vi "Probability Bar.vi"(7 "QuWire in":refnum<class "QuWire.lvclass">) -> (4 "Porababilities":dbl[](array[numeric]), 15 "Qubits n":i32)   [LabVIEW 2020]
uses:
  QuSim/QuWire/QuWire.lvclass
panel:
  out "Probability Bar Graph":cluster{i32[], dbl[]}(graph)
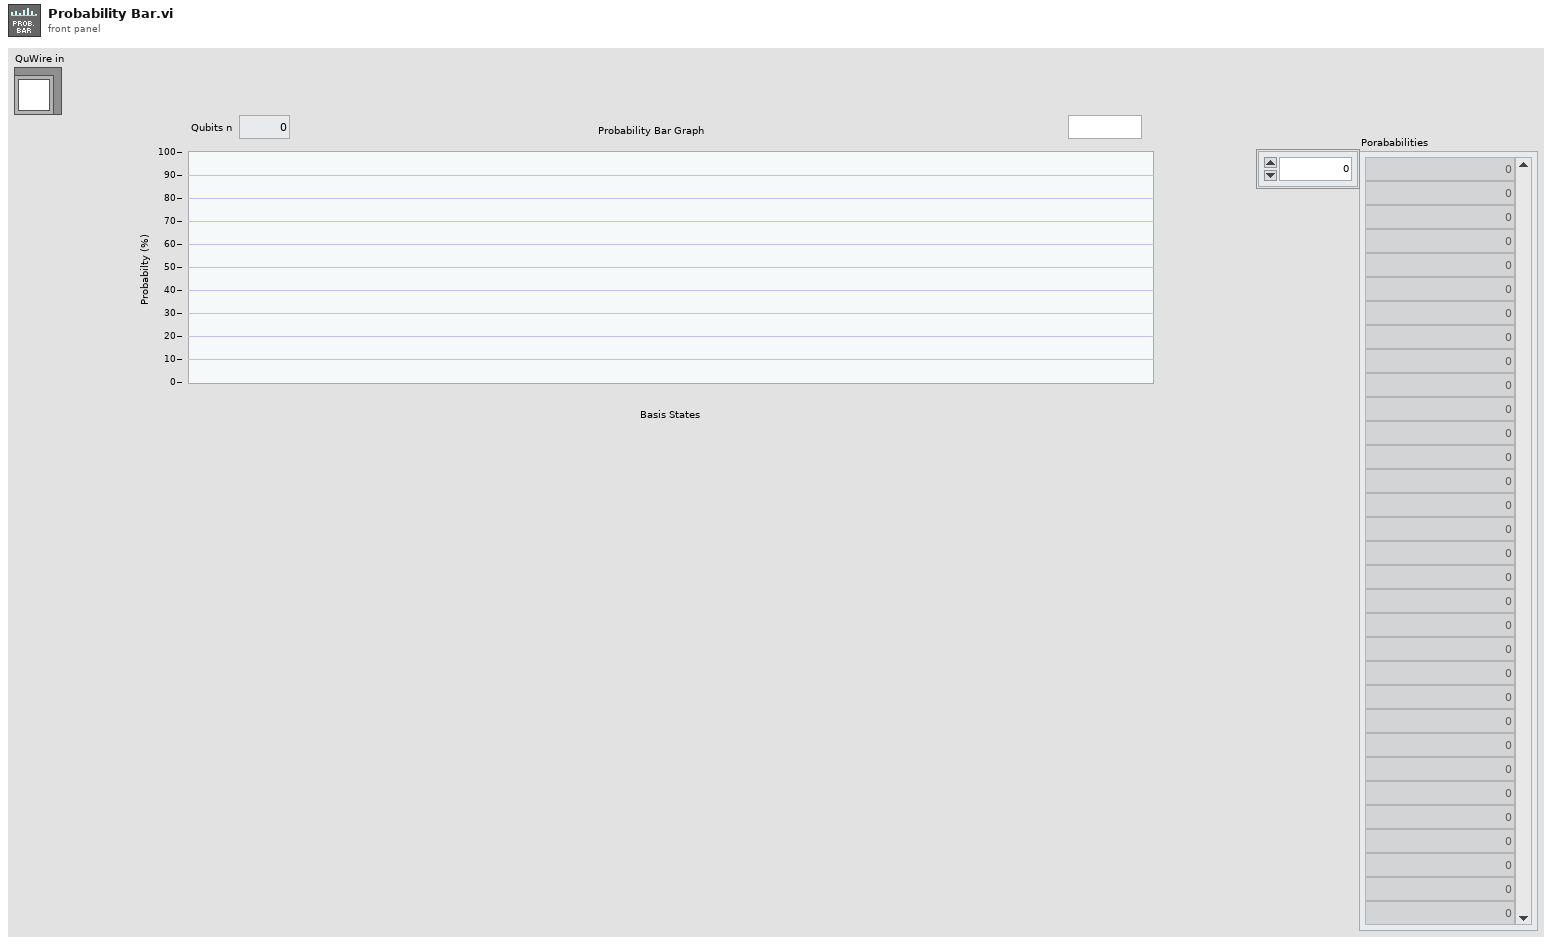
[diagram p1: front panel]
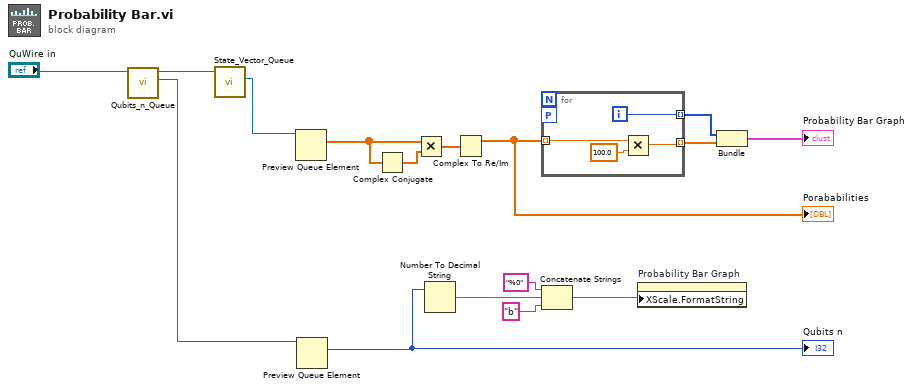
[diagram p0: block diagram]
diagram:
  n1 = call "Qubits_n_Queue.vi"("QuWire in"="QuWire in") -> ("Qubit n"=w10:refnum<queue>, "QuWire out"=w12:refnum<class "QuWire.lvclass">)  [unwired: 8 in, 1 out]
  n2 = call "State_Vector_Queue.vi"("QuWire in"=w12) -> ("State Vector Queue"=w16:refnum<queue>)  [unwired: 8 in, 2 out]
  n3 = Preview Queue Element(queue=w16) -> (element=w14:cdb[])  [unwired: 2 in, 3 out]
  n4 = Preview Queue Element(queue=w10) -> (element=w6:i32)  [unwired: 2 in, 3 out]
  "Qubits n" <- w6
  n5 = Complex Conjugate(1:w14) -> (0:w15:cdb[])
  n6 = Multiply(x=w14, y=w15) -> (x*y=w13:cdb[])
  n7 = Number To Decimal String(number=w6) -> (decimal integer string=w7:string)  [unwired: 1 in]
  n8 = Complex To Re/Im(x + iy=w13) -> (x=w5:dbl[])  [unwired: 1 out]
  "Porababilities" <- w5
  n9 = for {
    tunnel: w5 -> [w18] mode=indexing
    workers-P: _ -> [_]
    tunnel: [w20] -> w3 mode=indexing
    tunnel: [w17] -> w2 mode=indexing
    i -> [w20]
    n10 = Multiply(x=w18, y=100.0) -> (x*y=w17:dbl)
  }
  n11 = Concatenate Strings("%0" ("string"), w7, "b" ("string")) -> (w1:string)
  n12 = property on="Probability Bar Graph" class="XYGraph (strict)"("XScale.FormatString"=w1) -> ()  [unwired: 2 in, 2 out]
  n13 = Bundle(w3, w2) -> (→"Probability Bar Graph":cluster{i32[], dbl[]})  [unwired: 1 in]
